vi "Send Receive.vi"() -> ()   [LabVIEW 2011, in "LVH-EZ430.lvlib"]
uses:
  <vilib>/LabVIEW Hacker/LabVIEW Interface for EZ430-Chronos/LVH-EZ430.lvlib
  <vilib>/LabVIEW Hacker/LabVIEW Interface for EZ430-Chronos/Private/Type Defs/EZ430-Chronos Ref.ctl
panel:
  in  "Bytes To Read":u32=7
  out "EZ430-Chronos Config":T1
  in  "EZ430-Chronos Config 2":T1
  out "Error Out":errorcluster
  in  "Error In":errorcluster
  in  "Data":u8[](array[numeric])
  in  "Command":u8
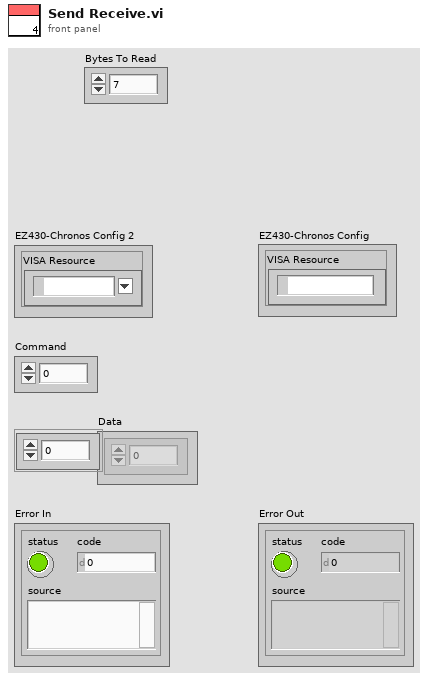
[diagram p1: front panel]
types:
  T1 = typedef "LVH-EZ430.lvlib/EZ430-Chronos Ref.ctl" = cluster{"VISA Resource":refnum<visa-resource-name>}
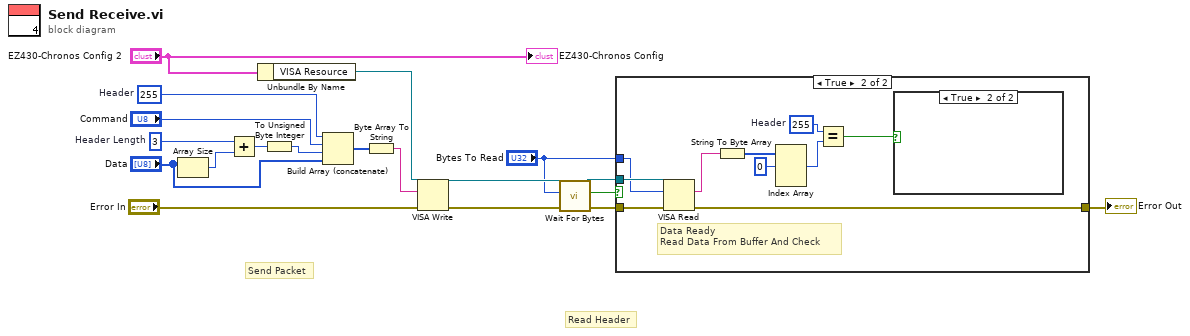
[diagram p0: block diagram]
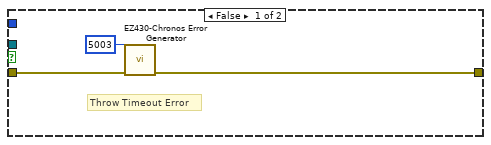
[diagram p2: hidden frame]
diagram:
  w16 = 3  # Header Length
  w19 = u8 255  # Header
  # "Read Header"
  # "Send Packet"
  n1 = Array Size(array="Data") -> (size(s)=w17:i32)
  n2 = Add(x=w16, y=w17) -> (x+y=w15:i32)
  n3 = Unbundle By Name("EZ430-Chronos Config 2") -> ("VISA Resource"=w11:refnum<visa-resource-name>)
  n4 = To Unsigned Byte Integer(number=w15) -> (unsigned 8bit integer=w14:u8)
  n5 = Build Array (concatenate)(w19, "Command", w14, "Data") -> (w12:u8[])
  n6 = Byte Array To String(unsigned byte array=w12) -> (string=w10:string)
  n7 = VISA Write(VISA resource name=w11, write buffer=w10, error in (no error)="Error In") -> (VISA resource name out=w6:refnum<visa-resource-name>, error out=w7:errorcluster)  [unwired: 1 out]
  n8 = call <vilib>:"Wait For Bytes.vi"("Error In"=w7, "Bytes To Read"="Bytes To Read", "VISA resource name"=w6) -> ("Error Out"=w4:errorcluster, "Bytes Available?"=w5:bool, "VISA resource name"=w2:refnum<visa-resource-name>)  [unwired: 6 in]
  n9 = case shown="True" w5 {
    tunnel: w4 -> [w22 w32]
    tunnel: [w21 w31] -> w3
    tunnel: w2 -> [_ w30]
    tunnel: "Bytes To Read" -> [_ w29]
    frame False {
      # "Throw Timeout Error"
      n10 = call <vilib>:"EZ430-Chronos Error Generator.vi"("Error In"=w22, "EZ430-Chronos Error Code"=5003) -> ("Error Out"=w21:errorcluster)  [unwired: 9 in]
    }
    frame True {
      w25 = u8 255  # Header
      # "Data Ready\nRead Data From Buffer And Check"
      n11 = VISA Read(VISA resource name=w30, byte count=w29, error in (no error)=w32) -> (read buffer=w28:string, error out=w31:errorcluster)  [unwired: 2 out]
      n12 = String To Byte Array(string=w28) -> (unsigned byte array=w27:u8[])
      n13 = Index Array(array=w27, index #1=0 ("index")) -> (element #1=w24:u8)  [unwired: 2 in, 2 out]
      n14 = Equal?(x=w25, y=w24) -> (x = y?=w23:bool)
      n15 = case shown="True" w23 {
        frame False {
        }
        frame True {
        }
      }
    }
  }
  "Error Out" <- w3
  "EZ430-Chronos Config" <- "EZ430-Chronos Config 2"
